vi "LowEnd.vi"() -> ()   [LabVIEW 2016, in "beamline sections.lvlib" / "Low energy end llb.lvlib"]
uses:
  low energy end/Low energy end/Low energy end llb.lvlib
  save load/saveloadprev.ctl
  save load/SaveLoad.lvlib
panel:
  in  "Tab Control":T1(tab)
  in  "Low Energy Einzel":dbl(slide) scale=0.0..50.0
  in  "Injector Image Einzel":dbl(slide) scale=0.0..50.0
  out "Low Energy Einzel Display":bool=TRUE
  out "Tank Entrance  Steerer Display":bool
  out "Low energy waist Steerer Display":bool=TRUE
  out "Injector Image Steerer display":bool
  out "Injector image Einzel Display":bool=TRUE
  in  "Tank Entrance Y2 steerer":dbl(slide) scale=-3.0..3.0
  in  "Tank Entrance Y1 steerer":dbl(slide) scale=-3.0..3.0
  in  "Tank Entrance  X steerer":dbl(slide) scale=-3.0..3.0
  in  "Low Energy Waist Y steerer":dbl(slide) scale=-3.0..3.0
  in  "Low Energy Waist  X steerer":dbl(slide) scale=-3.0..3.0
  in  "Injector Image Y steerer":dbl(slide) scale=-3.0..3.0
  in  "Injector Image X steerer":dbl(slide) scale=-3.0..3.0
  out "LE Einzel V":dbl format="%#.2g"
  out "LE Einzel I":dbl format="%#.2g"
  out "Tank Entrance X V read":dbl format="%#.2g"
  out "Tank Entrance Y1 V read":dbl format="%#.2g"
  out "Tank Entrance Y2 V read":dbl format="%#.2g"
  out "Low energy waist  X V":dbl format="%#.2g"
  out "Low energy waist  Y V":dbl format="%#.2g"
  out "Inj image Einzel I":dbl format="%#.2g"
  out "Inj image Einzel V":dbl format="%#.2g"
  out "Inj Image X Voltage":dbl format="%#.2g"
  out "Inj Image Y Voltage":dbl format="%#.2g"
  in  "stop":bool
  out "Tank entrance Ion gauge Cluster 1":T2
  out "LE Waist  Ion gauge Cluster":T2
  in  "Preview-Save-Load":T3
  out "LE Waist Steerer X+":dbl format="%#_4g"
  out "Tank Entrance X+ set":dbl format="%#_4g"
  out "Tank Entrance X- set":dbl format="%#_4g"
  out "Tank Entrance Y2+ set":dbl format="%#_4g"
  out "Tank Entrance Y2- set":dbl format="%#_4g"
  out "Tank Entrance Y1+ set":dbl format="%#_4g"
  out "Tank Entrance Y1- set":dbl format="%#_4g"
  out "Tank Entrance X- V read":dbl
  out "Tank Entrance Y1+ V read":dbl
  out "Tank Entrance Y2- V read":dbl
  out "Tank Entrance Y1- V read":dbl
  out "Tank Entrance Y2+ V read":dbl
  out "Tank Entrance X+ V read":dbl
  in  "LowEnd temp file":path=path "D:/Main Tune Parameters/Temp Configs/LowEnd.txt"
  out "SaveLoad error":errorcluster
  out "SV error - while loop":errorcluster
  out "SV error -event loop":errorcluster
  out "Low energy waist  X-":dbl format="%#_4g"
  out "Low energy waist  Y+":dbl format="%#_4g"
  out "Low energy waist  Y-":dbl format="%#_4g"
  # "Low Energy End"
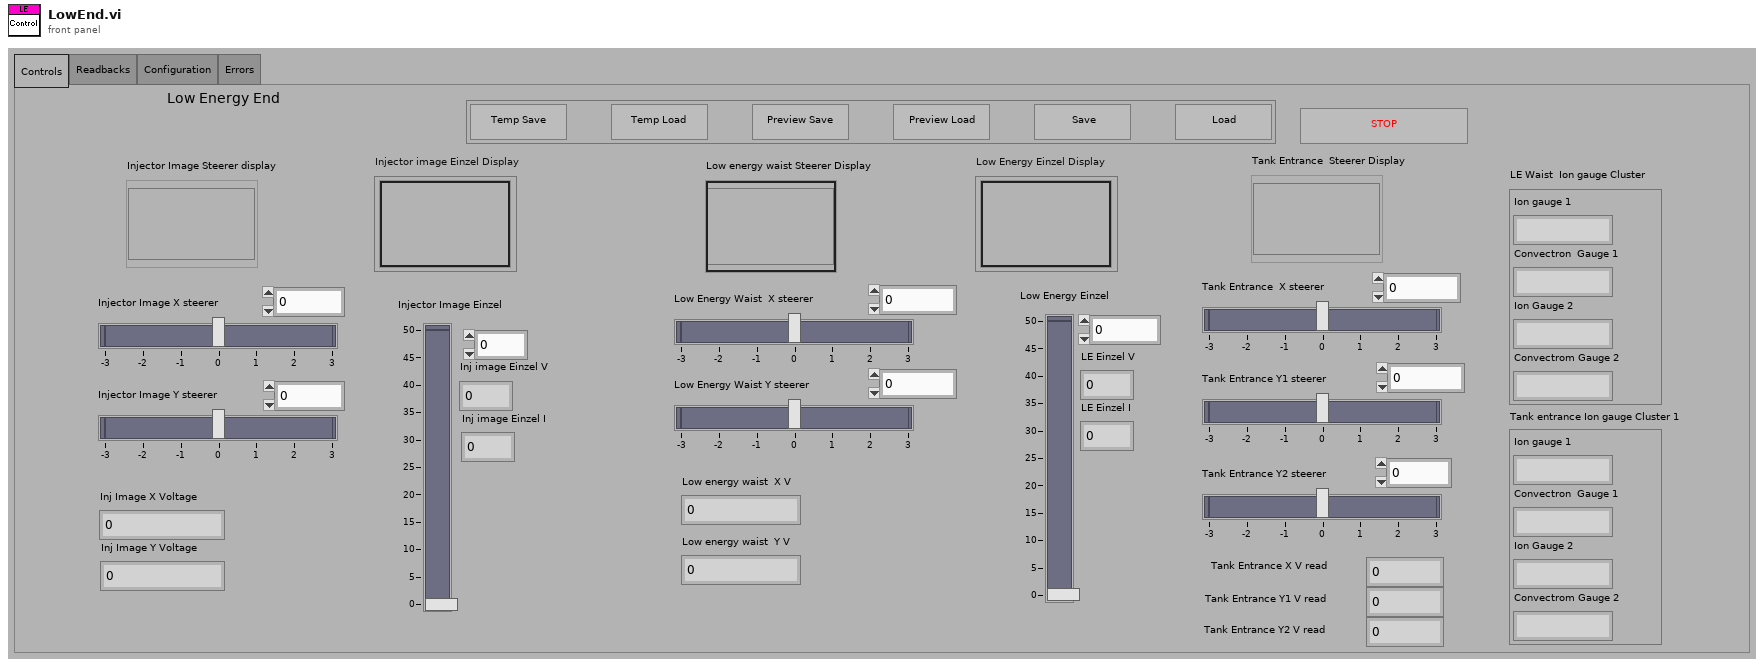
[diagram p1: front panel]
types:
  T1 = enum32{"Controls", "Readbacks", "Configuration", "Errors"}
  T2 = cluster{"Ion gauge 1":string, "Convectron  Gauge 1 ":string, "Ion Gauge 2":string, "Convectrom Gauge 2":string}
  T3 = typedef "saveloadprev.ctl" = cluster{"Temp Save":bool, "Temp Load":bool, "Save":bool, "Load":bool, "Preview Save":bool, "Preview Load":bool}
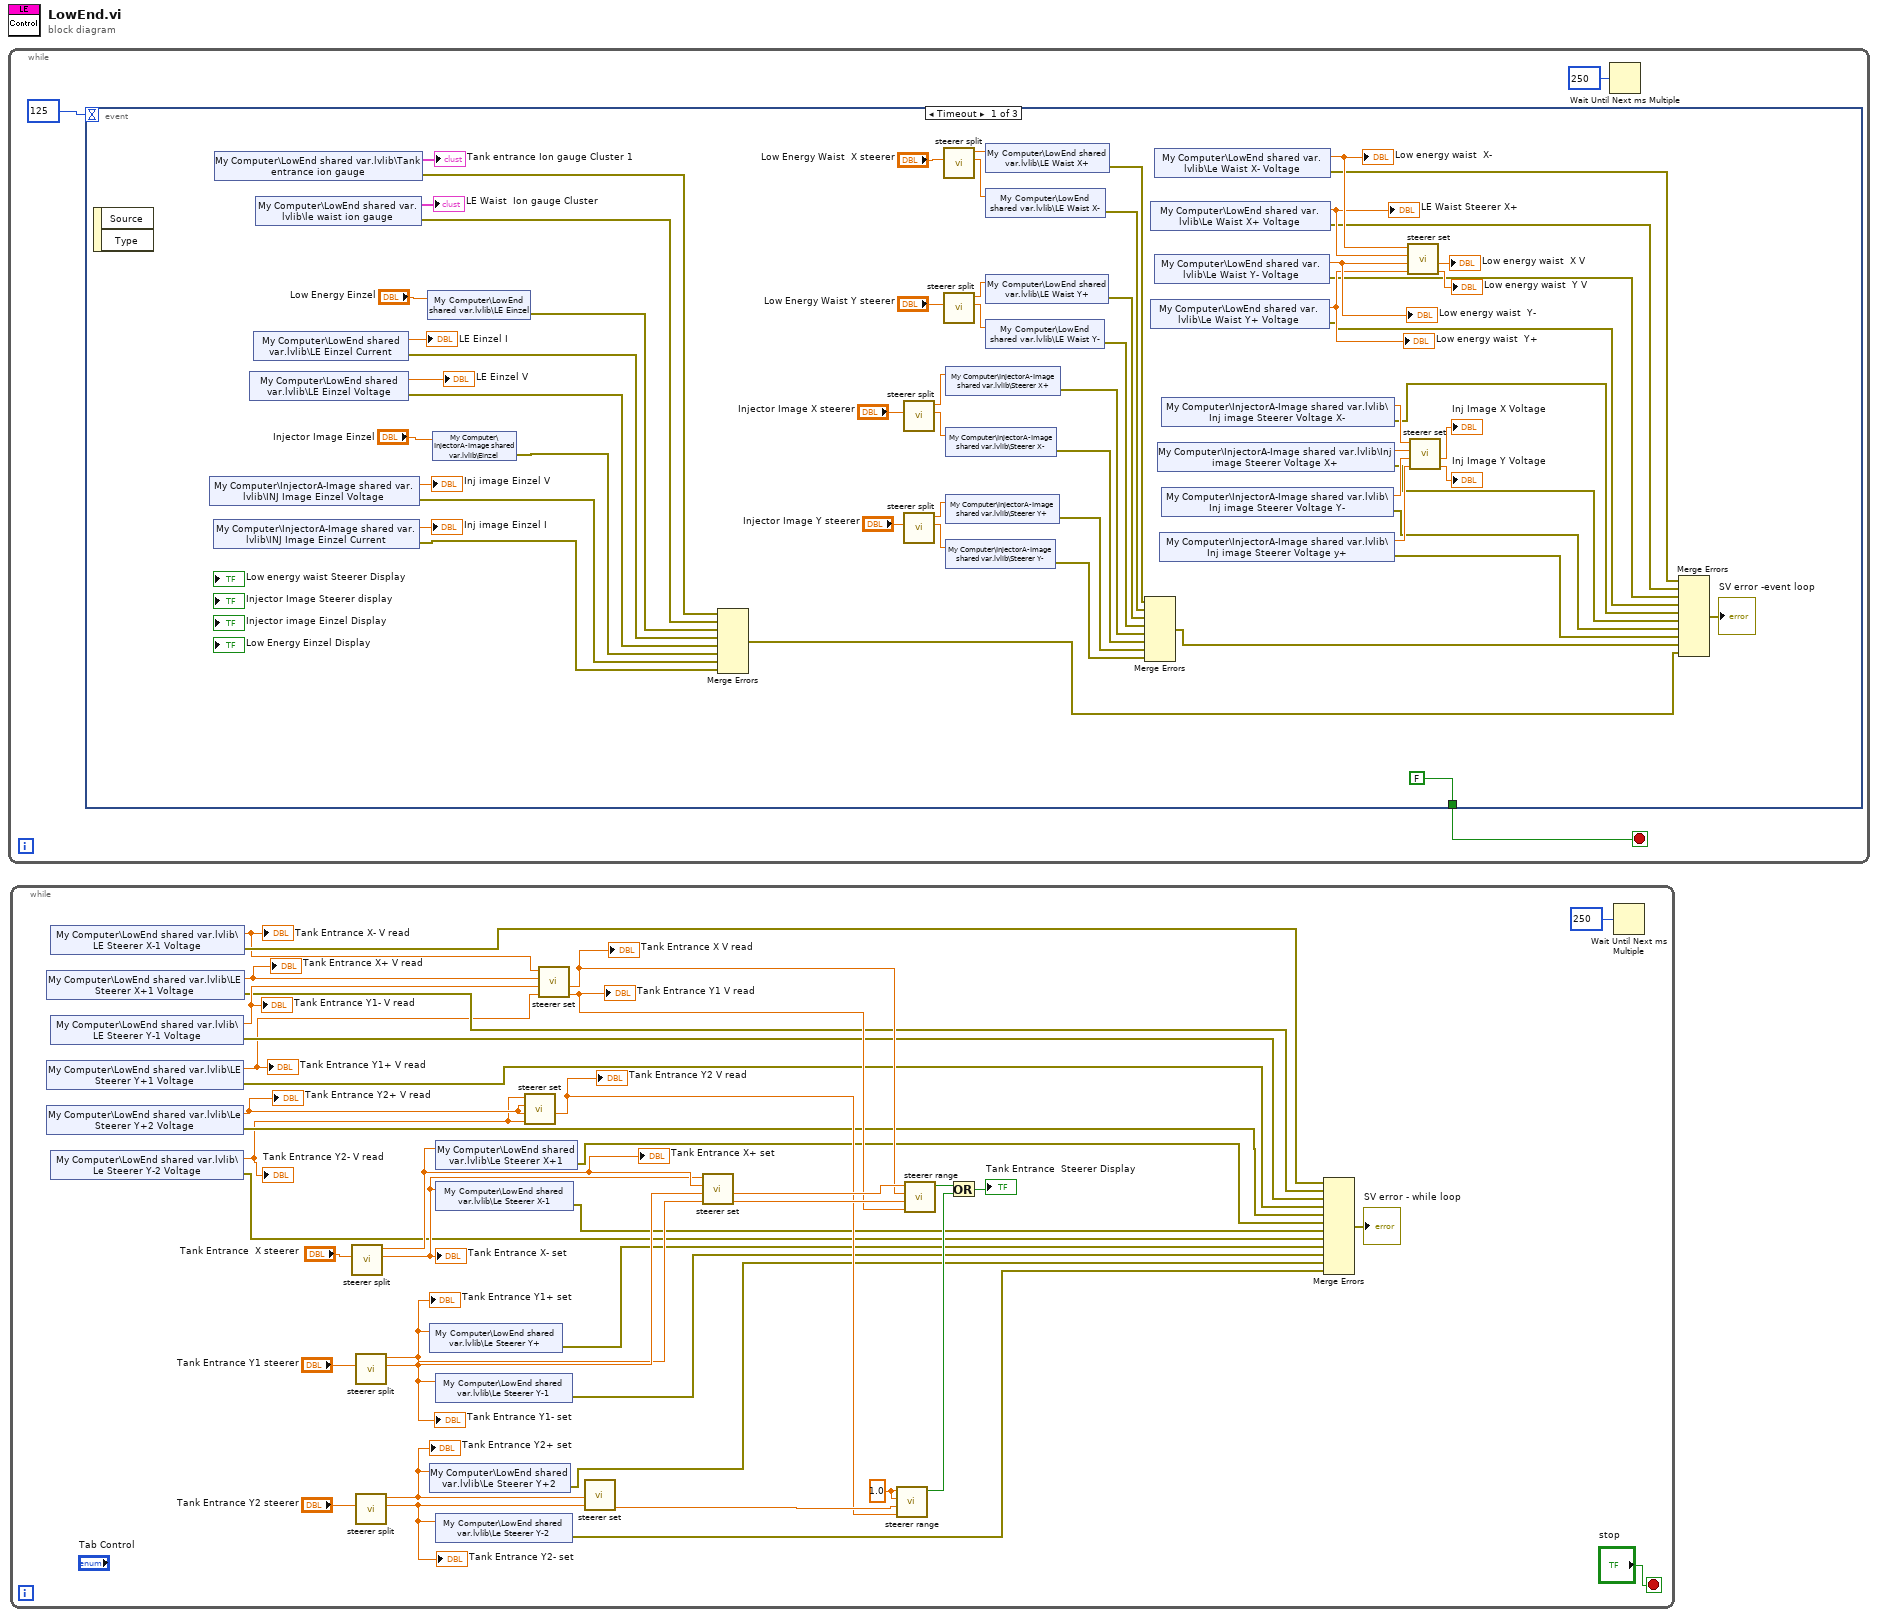
[diagram p0: block diagram]
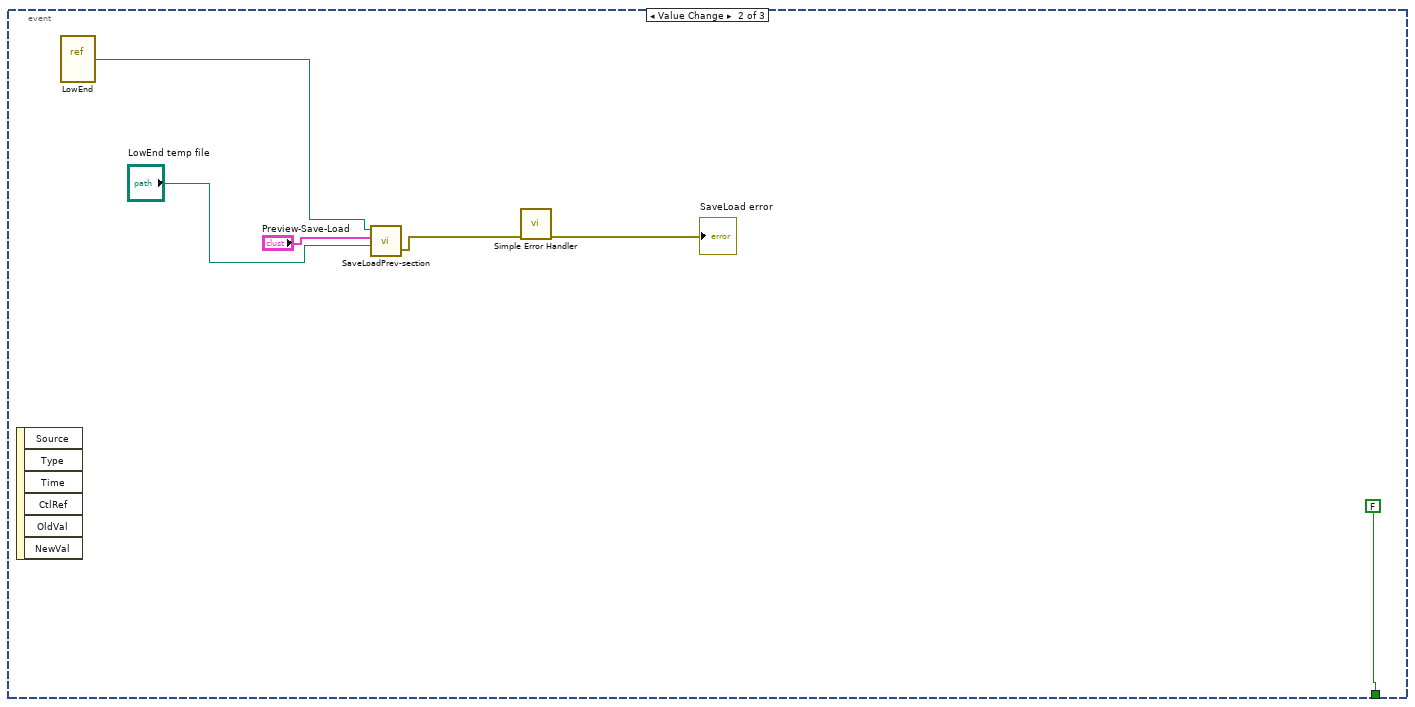
[diagram p2: hidden frame]
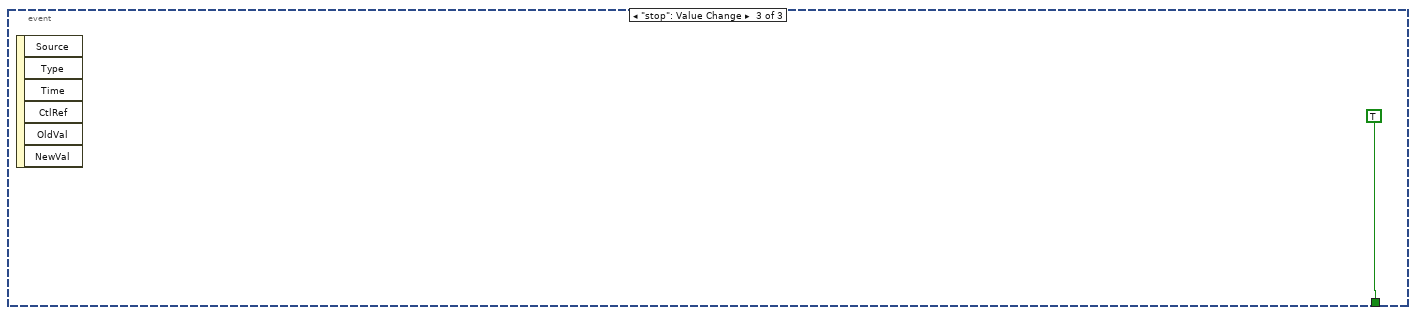
[diagram p3: hidden frame]
diagram:
  n1 = while {
    stop <- w2 stop-if-true
    n2 = event shown="[0] Timeout" {
      selector: _ -> [_ _ _]
      dyn-events: _ -> [_ _ _]
      timeout: 125 -> [_ _ _]
      tunnel: [FALSE FALSE TRUE] -> w2
      event Timeout {
        n3 = event-data() -> ()  [unwired: 1 in, 2 out]
        n4 = shared-variable "My Computer\\InjectorA-Image shared var.lvlib\\INJ Image Einzel Voltage"() -> (→"Inj image Einzel V":dbl, error out=w24:errorcluster)  [unwired: 1 in]
        n5 = shared-variable "My Computer\\InjectorA-Image shared var.lvlib\\INJ Image Einzel Current"() -> (→"Inj image Einzel I":dbl, error out=w23:errorcluster)  [unwired: 1 in]
        n6 = shared-variable "My Computer\\LowEnd shared var.lvlib\\Tank entrance ion gauge"() -> (→"Tank entrance Ion gauge Cluster 1":cluster{string, string, string, string}, error out=w30:errorcluster)  [unwired: 1 in]
        n7 = shared-variable "My Computer\\LowEnd shared var.lvlib\\LE Einzel Voltage"() -> (→"LE Einzel V":dbl, error out=w26:errorcluster)  [unwired: 1 in]
        n8 = shared-variable "My Computer\\LowEnd shared var.lvlib\\LE Einzel Current"() -> (→"LE Einzel I":dbl, error out=w27:errorcluster)  [unwired: 1 in]
        n9 = shared-variable "My Computer\\LowEnd shared var.lvlib\\le waist ion gauge"() -> (→"LE Waist  Ion gauge Cluster":cluster{string, string, string, string}, error out=w29:errorcluster)  [unwired: 1 in]
        n10 = shared-variable "My Computer\\LowEnd shared var.lvlib\\LE Einzel"("Low Energy Einzel") -> (error out=w28:errorcluster)  [unwired: 1 in]
        n11 = shared-variable "My Computer\\InjectorA-Image shared var.lvlib\\Einzel"("Injector Image Einzel") -> (error out=w25:errorcluster)  [unwired: 1 in]
        n12 = Merge Errors(w30, w29, w28, w27, w26, w25, w24, w23) -> (w5:errorcluster)
        n13 = call "steerer split.vi"("Steerer in"="Injector Image X steerer") -> ("Steerer +"=w37:dbl, "Steerer -"=w38:dbl)  [unwired: 7 out]
        n14 = call "steerer split.vi"("Steerer in"="Injector Image Y steerer") -> ("Steerer +"=w39:dbl, "Steerer -"=w40:dbl)  [unwired: 7 out]
        n15 = call "steerer split.vi"("Steerer in"="Low Energy Waist  X steerer") -> ("Steerer +"=w53:dbl, "Steerer -"=w54:dbl)  [unwired: 7 out]
        n16 = call "steerer split.vi"("Steerer in"="Low Energy Waist Y steerer") -> ("Steerer +"=w52:dbl, "Steerer -"=w51:dbl)  [unwired: 7 out]
        n17 = shared-variable "My Computer\\InjectorA-Image shared var.lvlib\\Steerer X+"(w37) -> (error out=w18:errorcluster)  [unwired: 1 in]
        n18 = shared-variable "My Computer\\InjectorA-Image shared var.lvlib\\Steerer X-"(w38) -> (error out=w17:errorcluster)  [unwired: 1 in]
        n19 = shared-variable "My Computer\\InjectorA-Image shared var.lvlib\\Steerer Y+"(w39) -> (error out=w16:errorcluster)  [unwired: 1 in]
        n20 = shared-variable "My Computer\\InjectorA-Image shared var.lvlib\\Steerer Y-"(w40) -> (error out=w15:errorcluster)  [unwired: 1 in]
        n21 = shared-variable "My Computer\\LowEnd shared var.lvlib\\LE Waist X+"(w53) -> (error out=w22:errorcluster)  [unwired: 1 in]
        n22 = shared-variable "My Computer\\LowEnd shared var.lvlib\\LE Waist X-"(w54) -> (error out=w21:errorcluster)  [unwired: 1 in]
        n23 = shared-variable "My Computer\\LowEnd shared var.lvlib\\LE Waist Y+"(w52) -> (error out=w20:errorcluster)  [unwired: 1 in]
        n24 = shared-variable "My Computer\\LowEnd shared var.lvlib\\LE Waist Y-"(w51) -> (error out=w19:errorcluster)  [unwired: 1 in]
        n25 = Merge Errors(w22, w21, w20, w19, w18, w17, w16, w15) -> (w6:errorcluster)
        n26 = shared-variable "My Computer\\LowEnd shared var.lvlib\\Le Waist X+ Voltage"() -> (w43:dbl, error out=w13:errorcluster)  [unwired: 1 in]
        "LE Waist Steerer X+" <- w43
        n27 = shared-variable "My Computer\\LowEnd shared var.lvlib\\Le Waist Y+ Voltage"() -> (w45:dbl, error out=w11:errorcluster)  [unwired: 1 in]
        "Low energy waist  Y+" <- w45
        n28 = shared-variable "My Computer\\LowEnd shared var.lvlib\\Le Waist X- Voltage"() -> (w44:dbl, error out=w14:errorcluster)  [unwired: 1 in]
        "Low energy waist  X-" <- w44
        n29 = shared-variable "My Computer\\LowEnd shared var.lvlib\\Le Waist Y- Voltage"() -> (w46:dbl, error out=w12:errorcluster)  [unwired: 1 in]
        "Low energy waist  Y-" <- w46
        n30 = shared-variable "My Computer\\InjectorA-Image shared var.lvlib\\Inj image Steerer Voltage X+"() -> (w34:dbl, error out=w9:errorcluster)  [unwired: 1 in]
        n31 = shared-variable "My Computer\\InjectorA-Image shared var.lvlib\\Inj image Steerer Voltage y+"() -> (w36:dbl, error out=w7:errorcluster)  [unwired: 1 in]
        n32 = shared-variable "My Computer\\InjectorA-Image shared var.lvlib\\Inj image Steerer Voltage X-"() -> (w35:dbl, error out=w10:errorcluster)  [unwired: 1 in]
        n33 = shared-variable "My Computer\\InjectorA-Image shared var.lvlib\\Inj image Steerer Voltage Y-"() -> (w33:dbl, error out=w8:errorcluster)  [unwired: 1 in]
        n34 = call "steerer set.vi"("Injector image X  -"=w44, "Injector image X +"=w43, "Injector image Y  -"=w46, "Injector image Y +"=w45) -> ("Steerer X"=→"Low energy waist  X V":dbl, "Steerer Y"=→"Low energy waist  Y V":dbl)  [unwired: 4 out]
        n35 = call "steerer set.vi"("Injector image X  -"=w35, "Injector image X +"=w34, "Injector image Y  -"=w33, "Injector image Y +"=w36) -> ("Steerer X"=→"Inj Image X Voltage":dbl, "Steerer Y"=→"Inj Image Y Voltage":dbl)  [unwired: 4 out]
        n36 = Merge Errors(w14, w13, w12, w11, w10, w9, w8, w7, w6, w5) -> (→"SV error -event loop":errorcluster)
      }
      event Value Change {
        n37 = event-data() -> ()  [unwired: 1 in, 6 out]
        n38 = vi-ref "LowEnd.vi"() -> (w66:refnum<vi>)
        n39 = call "SaveLoadPrev-section.vi"("file path (use dialog)"="LowEnd temp file", "Cluster 2"="Preview-Save-Load", "VI Refnum"=w66) -> ("error out"=w65:errorcluster)  [unwired: 2 in]
        n40 = call <vilib>:"Simple Error Handler.vi"("error in (no error)"=w65) -> ("error out"=→"SaveLoad error":errorcluster)  [unwired: 4 in, 4 out]
      }
      event "stop": Value Change {
        n41 = event-data() -> ()  [unwired: 1 in, 6 out]
      }
    }
    n42 = Wait Until Next ms Multiple(millisecond multiple=u32 250) -> ()  [unwired: 1 out]
  }
  n43 = while {
    stop <- "stop" stop-if-true
    w105 = 1.0 ("Steerer X Set")
    n44 = shared-variable "My Computer\\LowEnd shared var.lvlib\\LE Steerer X+1 Voltage"() -> (w72:dbl, error out=w86:errorcluster)  [unwired: 1 in]
    "Tank Entrance X+ V read" <- w72
    n45 = shared-variable "My Computer\\LowEnd shared var.lvlib\\LE Steerer Y+1 Voltage"() -> (w75:dbl, error out=w84:errorcluster)  [unwired: 1 in]
    "Tank Entrance Y1+ V read" <- w75
    n46 = shared-variable "My Computer\\LowEnd shared var.lvlib\\Le Steerer Y+2 Voltage"() -> (w97:dbl, error out=w83:errorcluster)  [unwired: 1 in]
    "Tank Entrance Y2+ V read" <- w97
    n47 = shared-variable "My Computer\\LowEnd shared var.lvlib\\LE Steerer X-1 Voltage"() -> (w73:dbl, error out=w87:errorcluster)  [unwired: 1 in]
    "Tank Entrance X- V read" <- w73
    n48 = shared-variable "My Computer\\LowEnd shared var.lvlib\\LE Steerer Y-1 Voltage"() -> (w98:dbl, error out=w85:errorcluster)  [unwired: 1 in]
    "Tank Entrance Y1- V read" <- w98
    n49 = shared-variable "My Computer\\LowEnd shared var.lvlib\\Le Steerer Y-2 Voltage"() -> (w74:dbl, error out=w80:errorcluster)  [unwired: 1 in]
    "Tank Entrance Y2- V read" <- w74
    n50 = call "steerer split.vi"("Steerer in"="Tank Entrance  X steerer") -> ("Steerer +"=w92:dbl, "Steerer -"=w91:dbl)  [unwired: 7 out]
    "Tank Entrance X+ set" <- w92
    "Tank Entrance X- set" <- w91
    n51 = call "steerer split.vi"("Steerer in"="Tank Entrance Y1 steerer") -> ("Steerer +"=w93:dbl, "Steerer -"=w94:dbl)  [unwired: 7 out]
    "Tank Entrance Y1+ set" <- w93
    "Tank Entrance Y1- set" <- w94
    n52 = call "steerer split.vi"("Steerer in"="Tank Entrance Y2 steerer") -> ("Steerer +"=w95:dbl, "Steerer -"=w96:dbl)  [unwired: 7 out]
    "Tank Entrance Y2+ set" <- w95
    "Tank Entrance Y2- set" <- w96
    n53 = shared-variable "My Computer\\LowEnd shared var.lvlib\\Le Steerer Y+"(w93) -> (error out=w79:errorcluster)  [unwired: 1 in]
    n54 = shared-variable "My Computer\\LowEnd shared var.lvlib\\Le Steerer Y+2"(w95) -> (error out=w71:errorcluster)  [unwired: 1 in]
    n55 = shared-variable "My Computer\\LowEnd shared var.lvlib\\Le Steerer X+1"(w92) -> (error out=w81:errorcluster)  [unwired: 1 in]
    n56 = shared-variable "My Computer\\LowEnd shared var.lvlib\\Le Steerer X-1"(w91) -> (error out=w82:errorcluster)  [unwired: 1 in]
    n57 = shared-variable "My Computer\\LowEnd shared var.lvlib\\Le Steerer Y-1"(w94) -> (error out=w78:errorcluster)  [unwired: 1 in]
    n58 = shared-variable "My Computer\\LowEnd shared var.lvlib\\Le Steerer Y-2"(w96) -> (error out=w77:errorcluster)  [unwired: 1 in]
    n59 = call "steerer set.vi"("Injector image X  -"=w74, "Injector image X +"=w97, "Injector image Y  -"=w97, "Injector image Y +"=w74) -> ("Steerer X"=w88:dbl)  [unwired: 5 out]
    "Tank Entrance Y2 V read" <- w88
    n60 = call "steerer set.vi"("Injector image X  -"=w73, "Injector image X +"=w72, "Injector image Y  -"=w98, "Injector image Y +"=w75) -> ("Steerer X"=w90:dbl, "Steerer Y"=w89:dbl)  [unwired: 4 out]
    "Tank Entrance X V read" <- w90
    "Tank Entrance Y1 V read" <- w89
    n61 = call "steerer set.vi"("Injector image Y  -"=w96, "Injector image Y +"=w95) -> ("Steerer Y"=w106:dbl)  [unwired: 2 in, 5 out]
    n62 = call "steerer set.vi"("Injector image X  -"=w91, "Injector image X +"=w92, "Injector image Y  -"=w94, "Injector image Y +"=w93) -> ("Steerer X"=w108:dbl, "Steerer Y"=w107:dbl)  [unwired: 4 out]
    n63 = call "steerer range.vi"("Steerer Y Voltage"=w88, "Steerer X Voltage"=w106, "Steerer Set Y"=w105, "Steerer X Set"=w105) -> ("Steerer within range"=w104:bool)  [unwired: 3 out]
    n64 = call "steerer range.vi"("Steerer Y Voltage"=w89, "Steerer X Voltage"=w107, "Steerer Set Y"=w90, "Steerer X Set"=w108) -> ("Steerer within range"=w103:bool)  [unwired: 3 out]
    n65 = Or(x=w103, y=w104) -> (x .or. y?=→"Tank Entrance  Steerer Display":bool)
    n66 = Merge Errors(w87, w86, w85, w84, w83, w81, w82, w80, w79, w78, w71, w77) -> (→"SV error - while loop":errorcluster)
    n67 = Wait Until Next ms Multiple(millisecond multiple=u32 250) -> ()  [unwired: 1 out]
  }
